vi "Write Vendor Name.vi"(8 "error in (no error)":errorcluster, 10 "vendor name":string, 11 "Asset in":refnum<class "Asset.lvclass">) -> (0 "error out":errorcluster, 3 "Asset out":refnum<class "Asset.lvclass">)   [LabVIEW 2018, in "Asset.lvclass"]
uses:
  Asset.lvclass
  Asset.lvclass/Asset.ctl
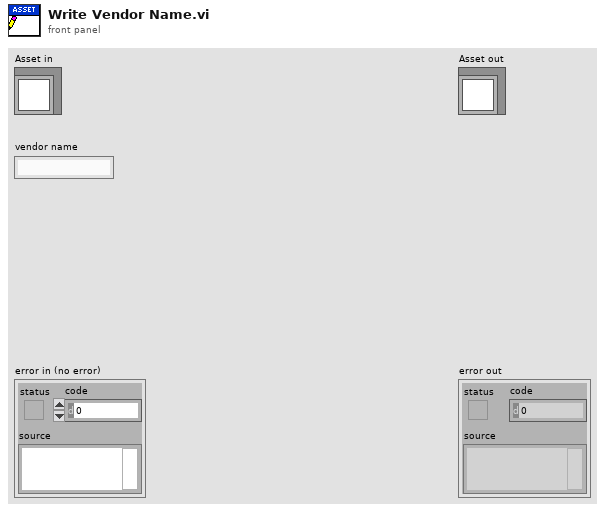
[diagram p1: front panel]
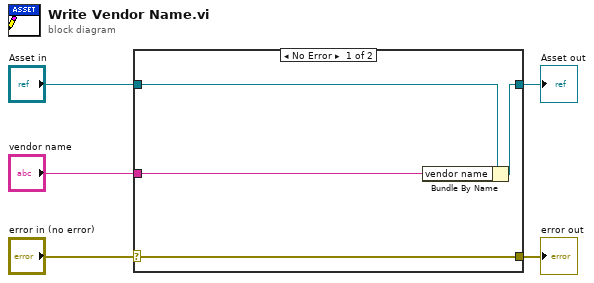
[diagram p0: block diagram]
diagram:
  n1 = case shown="No Error" "error in (no error)" {
    selector: "error in (no error)" -> [w9 w10]
    tunnel: [w9 w10] -> w4
    tunnel: [w7 w11] -> w2
    tunnel: "Asset in" -> [w8 w11]
    tunnel: "vendor name" -> [w6 _]
    frame No Error {
      n2 = Bundle By Name(cluster=w8, "vendor name"=w6) -> (w7:refnum<class "Asset.lvclass">)
    }
    frame Error {
    }
  }
  "error out" <- w4
  "Asset out" <- w2
